vi "Rectangle Sub-Parser.vi"(2 "error in (no error)":errorcluster, 3 "Transformation Matrix":T1, 4 "Array of Nodes":string[](array[string])) -> (0 "error out":errorcluster, 1 "rects":T2(array[cluster]))   [LabVIEW 2013]
uses:
  <vilib>/Analysis/Matrix/Datatypes/RealMatrix.ctl
  <vilib>/Analysis/baseanly.llb/Real A x B.vi
  <vilib>/Analysis/NI_AALBase.lvlib
  <vilib>/Analysis/Matrix/NI_Matrix.lvlib
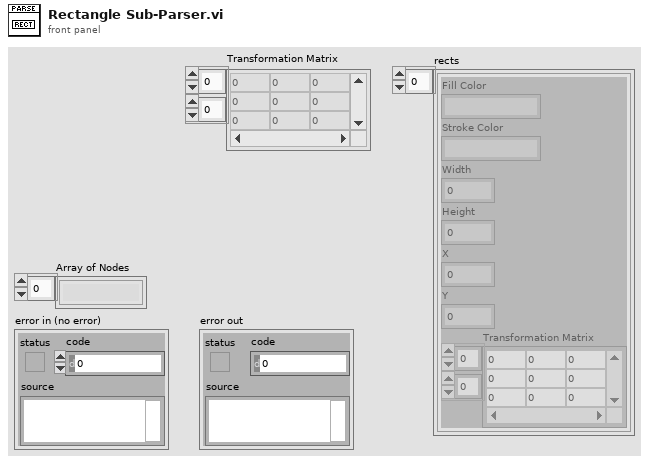
[diagram p1: front panel]
types:
  T1 = typedef "NI_Matrix.lvlib/RealMatrix.ctl" = dbl[][]
  T2 = cluster{"Fill Color":string, "Stroke Color":string, "Width":dbl, "Height":dbl, "X":dbl, "Y":dbl, "Transformation Matrix":T1}[]
  T3 = cluster{"XML":string, "XML":string, dbl, dbl, dbl, dbl, "Transformation Matrix":T1}
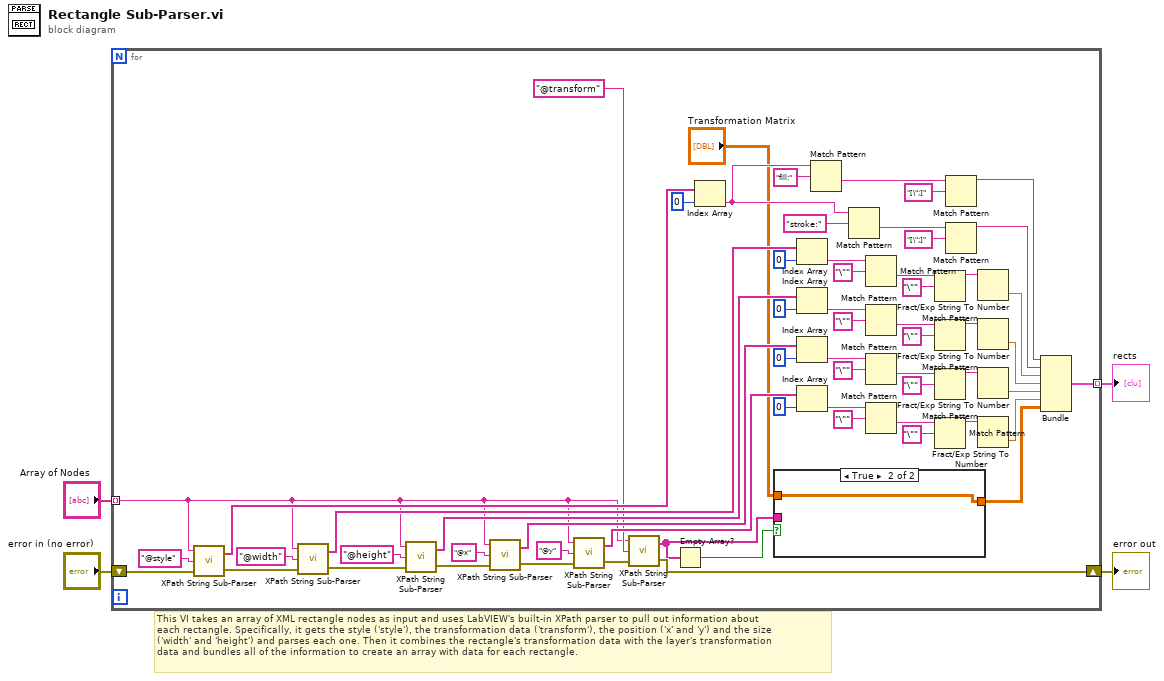
[diagram p0: block diagram]
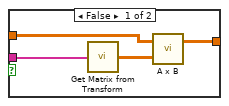
[diagram p2: hidden frame]
diagram:
  # "This VI takes an array of XML rectangle nodes as input and uses LabVIEW's built-in XPath parser to pull out information about \neach rectangle. Specifically, it gets the style ('style'), the transformation data ('transform'), the position ('x' and 'y') and the size \n('width' and 'height') and parses each one. Then it combines the rectangle's transformation data with the layer's transformation \ndata and bundles all of the information to create an array with data for each rectangle."
  n1 = for {
    tunnel: "Array of Nodes" -> [w9] mode=indexing
    shift-right: [w10] -> w2
    shift-left: "error in (no error)" -> [w59]
    tunnel: [w26] -> w1 mode=indexing
    n2 = call "XPath String Sub-Parser.vi"("error in (no error)"=w59, "XPath expression"="@style", "XML String"=w9) -> ("error out"=w58:errorcluster, "Array of Results"=w65:string[])
    n3 = call "XPath String Sub-Parser.vi"("error in (no error)"=w58, "XPath expression"="@width", "XML String"=w9) -> ("error out"=w57:errorcluster, "Array of Results"=w38:string[])
    n4 = call "XPath String Sub-Parser.vi"("error in (no error)"=w57, "XPath expression"="@height", "XML String"=w9) -> ("error out"=w56:errorcluster, "Array of Results"=w39:string[])
    n5 = call "XPath String Sub-Parser.vi"("error in (no error)"=w56, "XPath expression"="@x", "XML String"=w9) -> ("error out"=w35:errorcluster, "Array of Results"=w40:string[])
    n6 = call "XPath String Sub-Parser.vi"("error in (no error)"=w35, "XPath expression"="@y", "XML String"=w9) -> ("error out"=w11:errorcluster, "Array of Results"=w28:string[])
    n7 = call "XPath String Sub-Parser.vi"("error in (no error)"=w11, "XPath expression"="@transform", "XML String"=w9) -> ("error out"=w10:errorcluster, "Array of Results"=w7:string[])
    n8 = Empty Array?(array=w7) -> (empty?=w5:bool)
    n9 = Index Array(array=w65, index=0) -> (element=w16:string)
    n10 = case shown="True" w5 {
      tunnel: [w70 w71] -> w8
      tunnel: w7 -> [w68 _]
      tunnel: "Transformation Matrix" -> [w67 w71]
      frame False {
        n11 = call "Get Matrix from Transform.vi"("Transform Attributes"=w68) -> ("Matrix"=w69:T1)
        n12 = call-poly <vilib>:"A x B.vi"("B"=w69, "A"=w67) -> ("A x B"=w70:T1)  [unwired: 1 out]
      }
      frame True {
      }
    }
    n13 = Index Array(array=w38, index=0) -> (element=w52:string)
    n14 = Index Array(array=w39, index=0) -> (element=w49:string)
    n15 = Index Array(array=w40, index=0) -> (element=w42:string)
    n16 = Index Array(array=w28, index=0) -> (element=w32:string)
    n17 = Match Pattern(string=w16, regular expression="fill:") -> (after substring=w62:string)  [unwired: 1 in, 3 out]
    n18 = Match Pattern(string=w16, regular expression="stroke:") -> (after substring=w17:string)  [unwired: 1 in, 3 out]
    n19 = Match Pattern(string=w52, regular expression="\"") -> (after substring=w54:string)  [unwired: 1 in, 3 out]
    n20 = Match Pattern(string=w49, regular expression="\"") -> (after substring=w47:string)  [unwired: 1 in, 3 out]
    n21 = Match Pattern(string=w42, regular expression="\"") -> (after substring=w44:string)  [unwired: 1 in, 3 out]
    n22 = Match Pattern(string=w32, regular expression="\"") -> (after substring=w30:string)  [unwired: 1 in, 3 out]
    n23 = Match Pattern(string=w54, regular expression="\"") -> (before substring=w23:string)  [unwired: 1 in, 3 out]
    n24 = Match Pattern(string=w47, regular expression="\"") -> (before substring=w24:string)  [unwired: 1 in, 3 out]
    n25 = Match Pattern(string=w44, regular expression="\"") -> (before substring=w25:string)  [unwired: 1 in, 3 out]
    n26 = Match Pattern(string=w30, regular expression="\"") -> (before substring=w27:string)  [unwired: 1 in, 3 out]
    n27 = Match Pattern(string=w62, regular expression="[\";]") -> (before substring=w14:string)  [unwired: 1 in, 3 out]
    n28 = Match Pattern(string=w17, regular expression="[\";]") -> (before substring=w13:string)  [unwired: 1 in, 3 out]
    n29 = Fract/Exp String To Number(string=w23) -> (number=w22:dbl)  [unwired: 3 in, 1 out]
    n30 = Fract/Exp String To Number(string=w24) -> (number=w21:dbl)  [unwired: 3 in, 1 out]
    n31 = Fract/Exp String To Number(string=w25) -> (number=w20:dbl)  [unwired: 3 in, 1 out]
    n32 = Fract/Exp String To Number(string=w27) -> (number=w19:dbl)  [unwired: 3 in, 1 out]
    n33 = Bundle("XML"=w14, "XML"=w13, w22, w21, w20, w19, "Transformation Matrix"=w8) -> (w26:T3)  [unwired: 1 in]
  }
  "error out" <- w2
  "rects" <- w1
